vi "层叠移位寄存器.vi"() -> ()   [LabVIEW 2015]
panel:
  in  "stop":bool
  out "当前值":dbl
  out "前三次循环":dbl
  out "前两次循环":dbl
  out "前一次循环":dbl
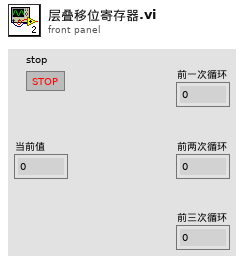
[diagram p1: front panel]
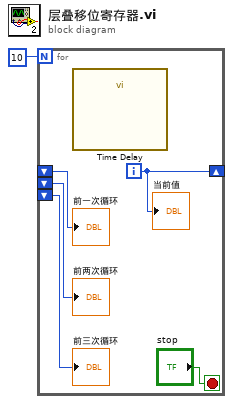
[diagram p0: block diagram]
diagram:
  n1 = for {
    N: 10 -> [_]
    shift-right: [w6] -> _
    shift-left: _ -> [w5]
    shift-left: _ -> [w4]
    shift-left: _ -> [w3]
    i -> [w6]
    stop <- "stop" stop-if-true
    n2 = call "Time Delay"() -> ()  [unwired: 11 in, 1 out]
    "前一次循环" <- w5
    "前两次循环" <- w4
    "前三次循环" <- w3
    "当前值" <- w6
  }
